vi "CanAttach.vi"(1 "Board":i32[][](array[numeric])=[[-3, -5, -4, -1, -2, -4, -5, -3], [-6, -6, -6, -6, -6, -6, -6, -6], [0, 0, 0, 0, 0, 0, 0, 0], [0, 0, 0, 0, 0, 0, 0, 0], [0, 0, 0, 0, 0, 0, 0, 0], [0, 0, 0, 0, 0, 0, 0, 0], [6, 6, 6, 6, 6, 6, 6, 6], [3, 5, 4, 1, 2, 4, 5, 3]], 2 "Black/White Turn (T/F)":bool, 3 "Column":i32, 4 "Row":i32) -> (0 "Boolean":bool)   [LabVIEW 2014]
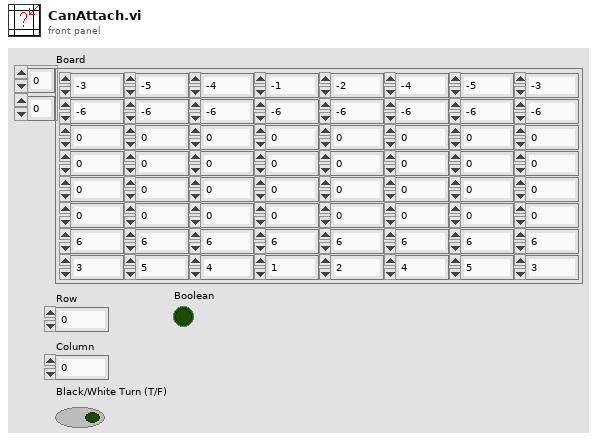
[diagram p1: front panel]
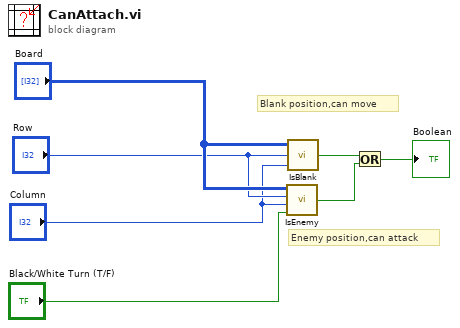
[diagram p0: block diagram]
diagram:
  # "Enemy position,can attack"
  # "Blank position,can move"
  n1 = call "IsEnemy.vi"("Black/White Turn (T/F)"="Black/White Turn (T/F)", "Column"="Column", "Row"="Row", "Board"="Board") -> ("Boolean"=w1:bool)
  n2 = call "IsBlank.vi"("Column"="Column", "Row"="Row", "Board"="Board") -> ("Boolean"=w6:bool)
  n3 = Or(x=w6, y=w1) -> (x .or. y?=→"Boolean":bool)
